vi "Get String Array Package Attribute Value.vi"(8 "error in (no error)":errorcluster, 10 "Package attribute name":string, 11 "package attributes CLI string":string) -> (0 "error out":errorcluster, 1 "attribute found?":bool, 3 "package attribute value":string[](array[string]))   [LabVIEW 2014, in "NIPM_API.lvlib"]
uses:
  NIPM_API.lvlib
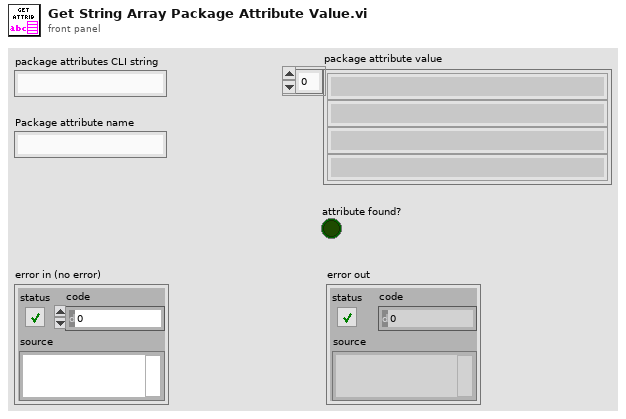
[diagram p1: front panel]
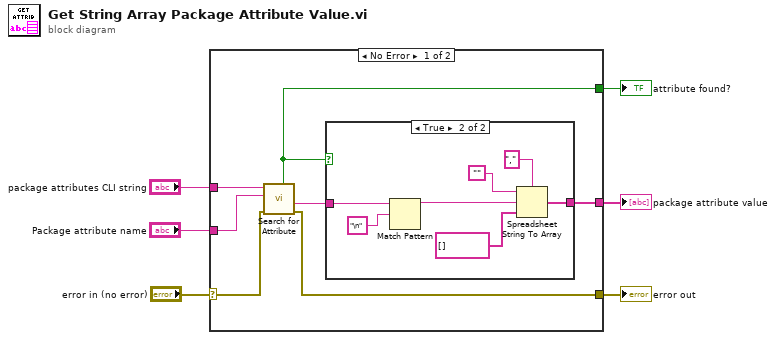
[diagram p0: block diagram]
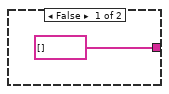
[diagram p2: hidden frame]
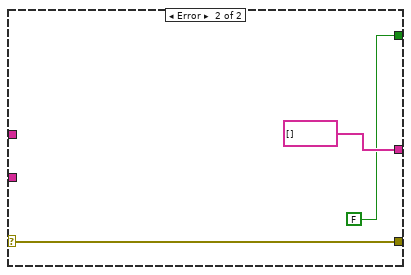
[diagram p3: hidden frame]
diagram:
  n1 = case shown="No Error" "error in (no error)" {
    selector: "error in (no error)" -> [w10 w24]
    tunnel: "Package attribute name" -> [w11 _]
    tunnel: "package attributes CLI string" -> [w12 _]
    tunnel: [w13 string[] [] ("Package Attribute Value")] -> w4
    tunnel: [w9 w24] -> w2
    tunnel: [w8 FALSE ("attribute found?")] -> w1
    frame No Error {
      n2 = call "Search for Attribute.vi"("error in (no error)"=w10, "package attribute name"=w11, "package attributes CLI string in"=w12) -> ("error out"=w9:errorcluster, "string after attribute"=w7:string, "attribute found?"=w8:bool)  [unwired: 3 in, 3 out]
      n3 = case shown="True" w8 {
        tunnel: [string[] [] ("Package Attribute Value") w18] -> w13
        tunnel: w7 -> [_ w15]
        frame False {
        }
        frame True {
          n4 = Match Pattern(string=w15, regular expression="\n") -> (before substring=w16:string)  [unwired: 1 in, 3 out]
          n5 = Spreadsheet String To Array(delimiter (Tab)=",", format string="", spreadsheet string=w16, array type (2D Dbl)=string[] [] ("Package Attribute Value")) -> (array=w18:string[])
        }
      }
    }
    frame Error {
    }
  }
  "package attribute value" <- w4
  "error out" <- w2
  "attribute found?" <- w1
